vi "Main.vi"() -> ()   [LabVIEW 2021]
uses:
  <vilib>/Utility/file.llb/Write Delimited Spreadsheet (string).vi
panel:
  in  "Stop":bool
  in  "file path":path
  out "Game State":enum16{"Easy", "med", "hard", "over"}(ring)
  out "Difficulty":enum16{"Easy", "Medium", "Hard"}(ring)
  in  "Start?":bool
  # "Start the Game ?"
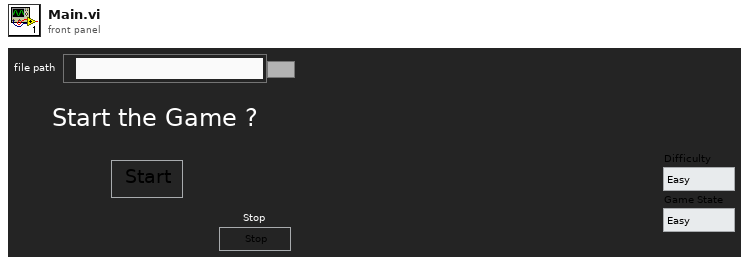
[diagram p1: front panel]
types:
  T1 = enum16{"Initialize", "Difficulty", "Start", "End"}
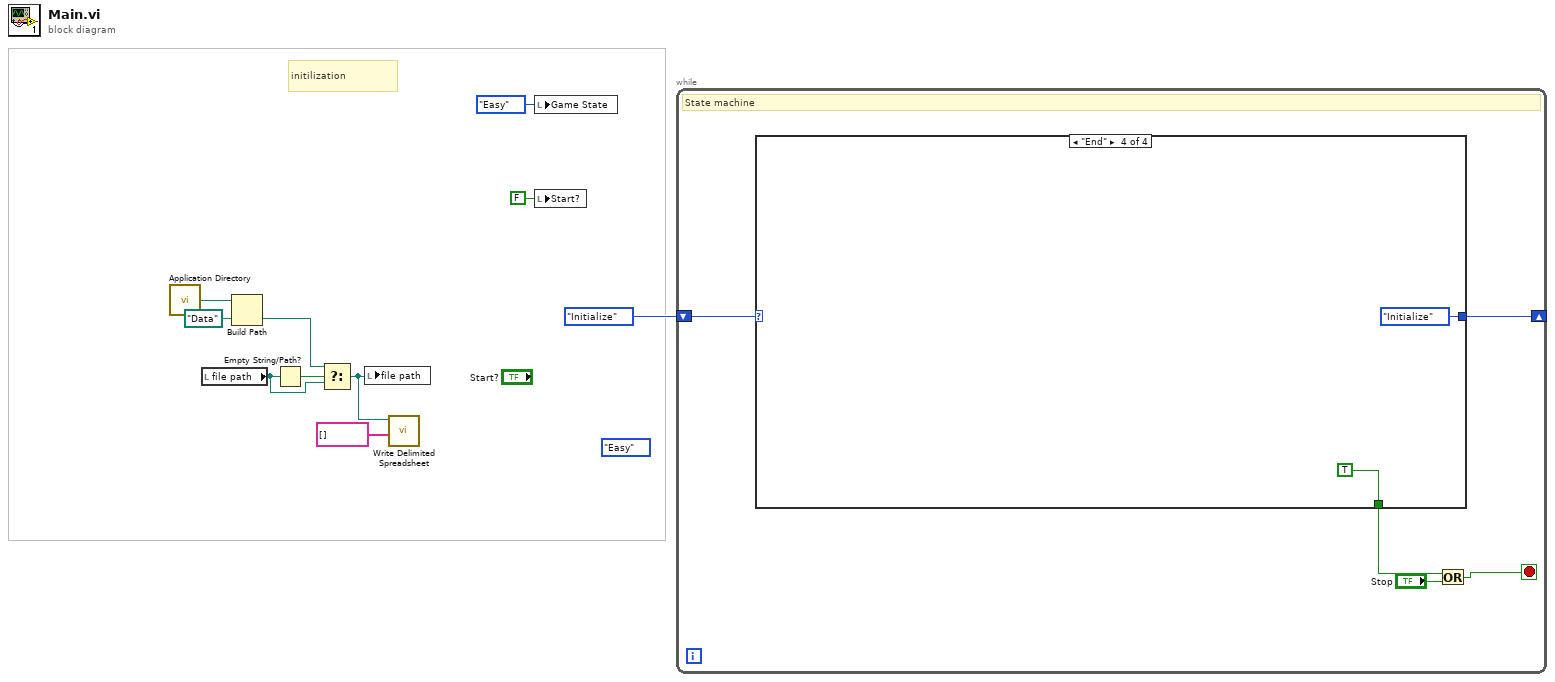
[diagram p0: block diagram]
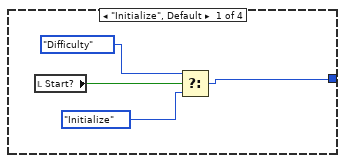
[diagram p2: hidden frame]
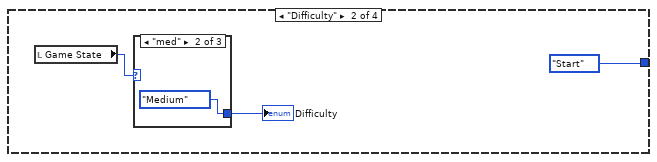
[diagram p3: hidden frame]
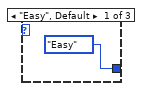
[diagram p4: hidden frame]
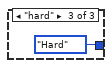
[diagram p5: hidden frame]
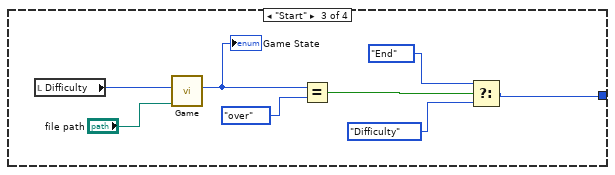
[diagram p6: hidden frame]
diagram:
  (unwired) enum16{"Easy", "Medium", "Hard"}."Easy"
  # "initilization"
  n1 = call <vilib>:"Application Directory.vi"() -> ("Application Directory"=w4:path)
  n2 = local read "file path"() -> (w6:path)
  n3 = Build Path(base path=w4, name or relative path=path "Data") -> (appended path=w5:path)
  n4 = Empty String/Path?(string/path=w6) -> (empty?=w7:bool)
  n5 = Select(t=w5, s=w7, f=w6) -> (s? t:f=w2:path)
  n6 = local write "file path"(w2) -> ()
  n7 = call-poly <vilib>:"Write Delimited Spreadsheet.vi"("file path (dialog if empty)"=w2, "1D data"=string[] [] ("appended array")) -> ()  [unwired: 12 in, 2 out]
  n8 = local write "Game State"(enum16{"Easy", "med", "hard", "over"}."Easy" ("Game State")) -> ()
  n9 = local write "Start?"(FALSE ("Start?")) -> ()
  n10 = while {
    shift-right: [w14] -> _
    shift-left: T1."Initialize" -> [w15]
    stop <- w12 stop-if-true
    # "State machine"
    n11 = case shown="\"End\"" w15 {
      tunnel: [w16 T1."Start" w29 T1."Initialize" ("f")] -> w14
      tunnel: [_ _ _ TRUE] -> w13
      frame "Initialize", Default {
        n12 = local read "Start?"() -> (w19:bool)
        n13 = Select(t=T1."Difficulty", s=w19, f=T1."Initialize") -> (s? t:f=w16:T1)
      }
      frame "Difficulty" {
        n14 = local read "Game State"() -> (w21:enum16{"Easy", "med", "hard", "over"})
        n15 = case shown="\"med\"" w21 {
          tunnel: [enum16{"Easy", "Medium", "Hard"}."Easy" ("Difficulty") enum16{"Easy", "Medium", "Hard"}."Medium" ("Difficulty") enum16{"Easy", "Medium", "Hard"}."Hard" ("Difficulty")] -> w20
          frame "Easy", Default {
          }
          frame "med" {
          }
          frame "hard" {
          }
        }
        "Difficulty" <- w20
      }
      frame "Start" {
        n16 = local read "Difficulty"() -> (w33:enum16{"Easy", "Medium", "Hard"})
        n17 = call "Game.vi"("file path"="file path", "Difficulty"=w33) -> ("Game state"=w27:enum16{"Easy", "med", "hard", "over"})  [unwired: 9 in]
        "Game State" <- w27
        n18 = Equal?(x=w27, y=enum16{"Easy", "med", "hard", "over"}."over") -> (x = y?=w32:bool)
        n19 = Select(t=T1."End", s=w32, f=T1."Difficulty") -> (s? t:f=w29:T1)
      }
      frame "End" {
      }
    }
    n20 = Or(x=w13, y="Stop") -> (x .or. y?=w12:bool)
  }
